vi "Teleop.vi"(10 "Match Info":T3={"Autonomous Elapsed Seconds"=0.0, "TeleOp Elapsed Seconds"=0.0, "Disabled Elapsed Seconds"=0.0, "Visited Autonomous"=FALSE, "Visited TeleOp"=FALSE, "Visited Disabled"=FALSE, "Autonomous Settings"={"Autonomous Style"=enum."Independent", "VI Refnum"=refnum}}, 11 "Call Context":T4) -> ()   [LabVIEW 2018]
doc: "This VI is called for each TeleOp packet received from the DS where the robot is not disabled. It is often used to read from the joysticks and update I/O or to update setpoints for timed control loops. It should complete and return within 20 milliseconds or it may miss DS packets."
uses:
  <vilib>/Rock Robotics/WPI/DriverStation/WPI_DriverStationDerivedRobotMode.ctl
  <vilib>/Rock Robotics/WPI/DriverStation/WPI_DriverStationMatch Info.ctl
  <vilib>/Rock Robotics/WPI/Utilities/WPI_GetSetVariantRefNum.vi
  <vilib>/Rock Robotics/Network Tables/NT Write Numeric Array.vi
  <vilib>/Rock Robotics/Network Tables/NT Read Boolean.vi
  <vilib>/Rock Robotics/Network Tables/NT Read Number.vi
  Robot Global Data.vi
  <vilib>/Rock Robotics/Network Tables/NT Write Boolean Array.vi
  <vilib>/addons/control/pid/pid.llb/PID (DBL).vi
  <vilib>/addons/control/pid/pid.llb/PID (DBL Array).vi
  <vilib>/Rock Robotics/WPI/Solenoid/Deprecated/WPI_SolenoidSetBool.vi
  <vilib>/addons/control/pid/NI_PID_pid.lvlib
panel:
  out "Distance 2":dbl
  in  "PID gains 4":T1={"proportional gain (Kc)"=1.0, "integral time (Ti, min)"=0.01, "derivative time (Td, min)"=0.0} {"derivative time (Td, min)" format="%.3f"; "integral time (Ti, min)" format="%.3f"; "proportional gain (Kc)" format="%.3f"}
  out "Direction 4":bool
  in  "Boolean":bool
  in  "PID gains 8":T1={"proportional gain (Kc)"=0.25, "integral time (Ti, min)"=0.001, "derivative time (Td, min)"=0.0}
  in  "PID gains":T2(array[cluster])=[{"proportional gain (Kc)"=1.0, "integral time (Ti, min)"=0.01, "derivative time (Td, min)"=0.0}] {"derivative time (Td, min)" format="%.3f"; "integral time (Ti, min)" format="%.3f"; "proportional gain (Kc)" format="%.3f"}
  in  "PID gains 2":T1={"proportional gain (Kc)"=1.0, "integral time (Ti, min)"=0.01, "derivative time (Td, min)"=0.0} {"derivative time (Td, min)" format="%.3f"; "integral time (Ti, min)" format="%.3f"; "proportional gain (Kc)" format="%.3f"}
  out "Compressor Running":bool
  out "Enable":bool
  out "Sample Slider 0":dbl(slide) scale=0.0..5.0
  out "Sample Boolean 1":bool
  out "Sample Boolean 0":bool
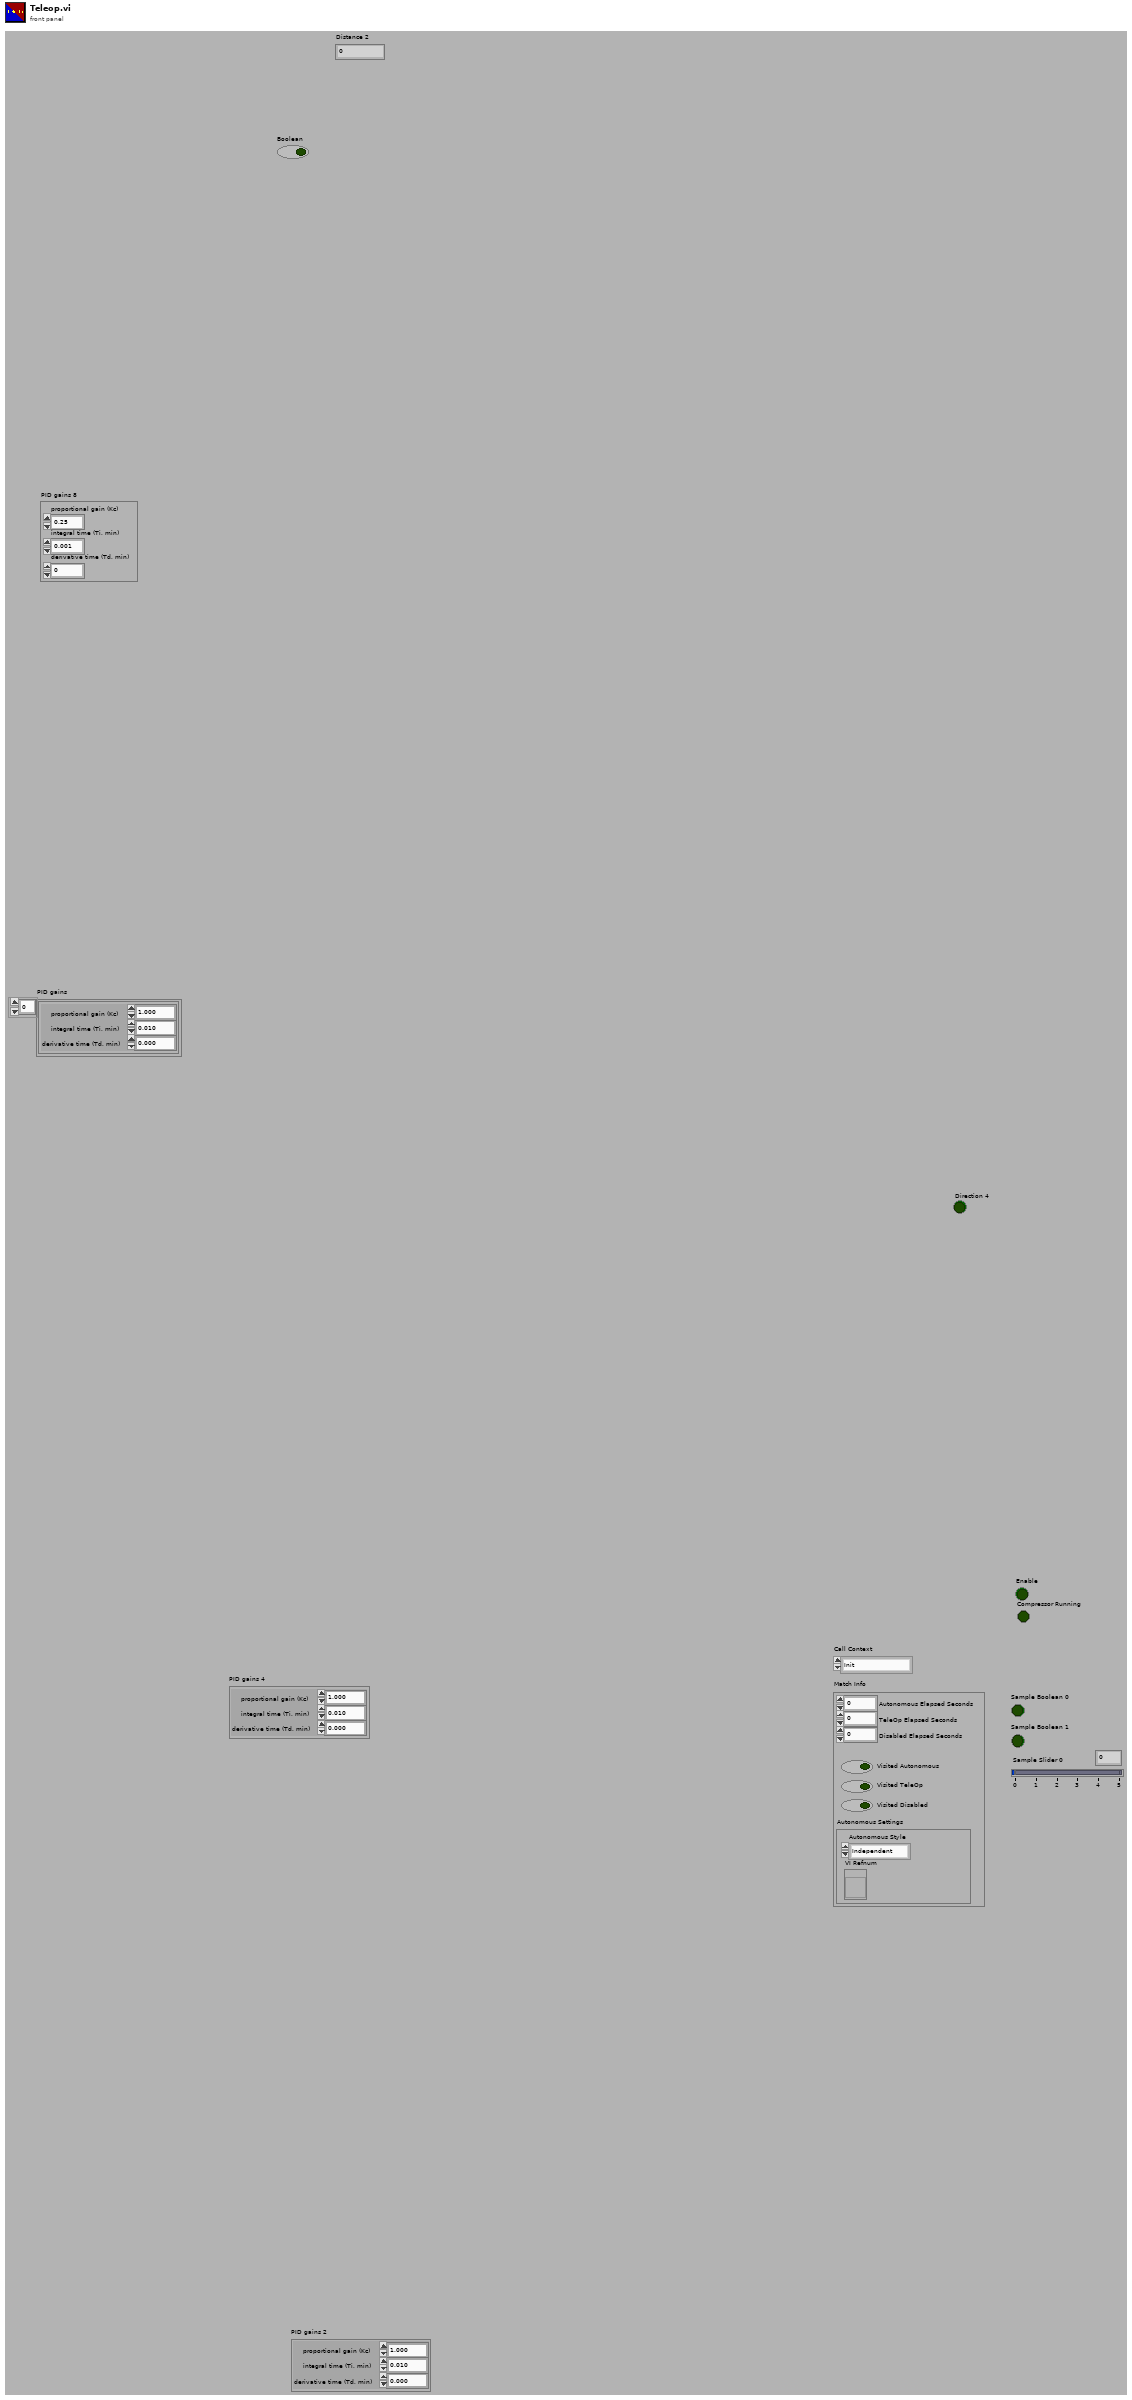
[diagram p1: front panel]
types:
  T1 = cluster{"proportional gain (Kc)":dbl, "integral time (Ti, min)":dbl, "derivative time (Td, min)":dbl}
  T2 = cluster{"proportional gain (Kc)":dbl, "integral time (Ti, min)":dbl, "derivative time (Td, min)":dbl}[]
  T3 = typedef "WPI_DriverStationMatch Info.ctl" = cluster{"Autonomous Elapsed Seconds":dbl, "TeleOp Elapsed Seconds":dbl, "Disabled Elapsed Seconds":dbl, "Visited Autonomous":bool, "Visited TeleOp":bool, "Visited Disabled":bool, "Autonomous Settings":cluster{"Autonomous Style":enum16{"Iterative", "Independent"}, "VI Refnum":refnum<vi>}}
  T4 = typedef "WPI_DriverStationDerivedRobotMode.ctl" = enum16{"Init", "Execute", "Stop"}
  T5 = enum16{"EXPULSA DISCO", "EXPULSA BOLA", "POSI敲O ENTREGA", "PEGAR BOLA", "POSI敲O NEUTRA", "DESCE ELEVADOR", "TERMINA SEQUENCIA"}[][]
  T6 = enum16{"EXPULSA DISCO", "EXPULSA BOLA", "POSI敲O ENTREGA", "PEGAR BOLA", "POSI敲O NEUTRA", "DESCE ELEVADOR", "TERMINA SEQUENCIA"}
  T7 = typedef "WPI_JoystickDevRef.ctl" = cluster{"Device":T8}
  T8 = typedef "WPI_JoystickDeviceEnum.ctl" = enum16{"USB 0", "USB 1", "USB 2", "USB 3", "USB 4", "USB 5"}
  T9 = typedef "WPI_EncoderDevRef.ctl" = cluster{"DevStatus":errorcluster, "EncoderIndex":T10, "CounterIndex":T11, "DistancePerCount":dbl, "Decoding Type":T12}
  T10 = typedef "FPGA_EncoderIdx.ctl" = enum8{"Enc 0", "Enc 1", "Enc 2", "Enc 3", "Enc 4", "Enc 5", "Enc 6", "Enc 7", "Invalid"}
  T11 = typedef "FPGA_CounterCtrSystemIndex.ctl" = enum8{"Ctr 0", "Ctr 1", "Ctr 2", "Ctr 3", "Ctr 4", "Ctr 5", "Ctr 6", "Ctr 7", "Invalid"}
  T12 = typedef "WPI_EncoderType.ctl" = enum16{"1x", "2x", "4x"}
  T13 = typedef "WPI_SolenoidDevRef.ctl" = cluster{"DevStatus":errorcluster, "Pneumatics Control Module":u8, "Forward Solenoid Channel":T14, "Reverse Solenoid Channel":T14}
  T14 = typedef "WPI_SolenoidChannel.ctl" = enum8{"Solenoid 0", "Solenoid 1", "Solenoid 2", "Solenoid 3", "Solenoid 4", "Solenoid 5", "Solenoid 6", "Solenoid 7", "Invalid"}
  T15 = typedef "WPI_DigitalInputDevRef.ctl" = cluster{"DevStatus":errorcluster, "DIO Channel":T16}
  T16 = typedef "FPGA_DIOChannel.ctl" = enum8{"DIO 0", "DIO 1", "DIO 2", "DIO 3", "DIO 4", "DIO 5", "DIO 6", "DIO 7", "DIO 8", "DIO 9", "DIO MXP 0", "DIO MXP 1", "DIO MXP 2", "DIO MXP 3", "DIO MXP 4", "DIO MXP 5", "DIO MXP 6", "DIO MXP 7", "DIO MXP 8", "DIO MXP 9", "DIO MXP 10", "DIO MXP 11", "DIO MXP 12", "DIO MXP 13", "DIO MXP 14", "DIO MXP 15", "SPI Port CS1", "SPI Port CS2", "SPI Port CS3", "SPI Port MISO", "SPI Port MOSI", "Invalid"}
  T17 = typedef "WPI_RobotDriveDevRef.ctl" = cluster{"DevStatus":errorcluster, "Motors[]":T18[], "Square Inputs":bool, "Max Output":dbl}
  T18 = typedef "WPI_MotorControlDeviceRef.ctl" = cluster{"DeviceStatus":errorcluster, "Type":T19, "PWM":cluster{"PWM Channel":T20, "DeadBand":T21}, "CAN":cluster{"Device Number":u8, "SetOutput VI Ref":variant, "GetOutput VI Ref":variant, "Enable VI Ref":variant, "Disable VI Ref":variant, "Data":variant}, "Invert":bool, "DIO PWM":cluster{"PWM \"Enable\" Channel":T20, "DIOChannel":T16, "PWM Rate":dbl}}
  T19 = typedef "WPI_MotorControlType.ctl" = enum16{"PWM", "CAN", "DIO PWM"}
  T20 = typedef "FPGA_DIOPWMChannel.ctl" = enum8{"PWM 0", "PWM 1", "PWM 2", "PWM 3", "PWM 4", "PWM 5", "PWM 6", "PWM 7", "PWM 8", "PWM 9", "PWM MXP 0", "PWM MXP 1", "PWM MXP 2", "PWM MXP 3", "PWM MXP 4", "PWM MXP 5", "PWM MXP 6", "PWM MXP 7", "PWM MXP 8", "PWM MXP 9", "Invalid"}
  T21 = typedef "WPI_PWMDeadband.ctl" = cluster{"Name":string, "maxPositivePwm":i32, "minPositivePwm":i32, "centerPwm":i32, "maxNegativePwm":i32, "minNegativePwm":i32, "angularRange":u16}
  T22 = typedef "WPI_CompressorDevRef.ctl" = cluster{"DevStatus":errorcluster, "Pneumatics Control Module":u8}
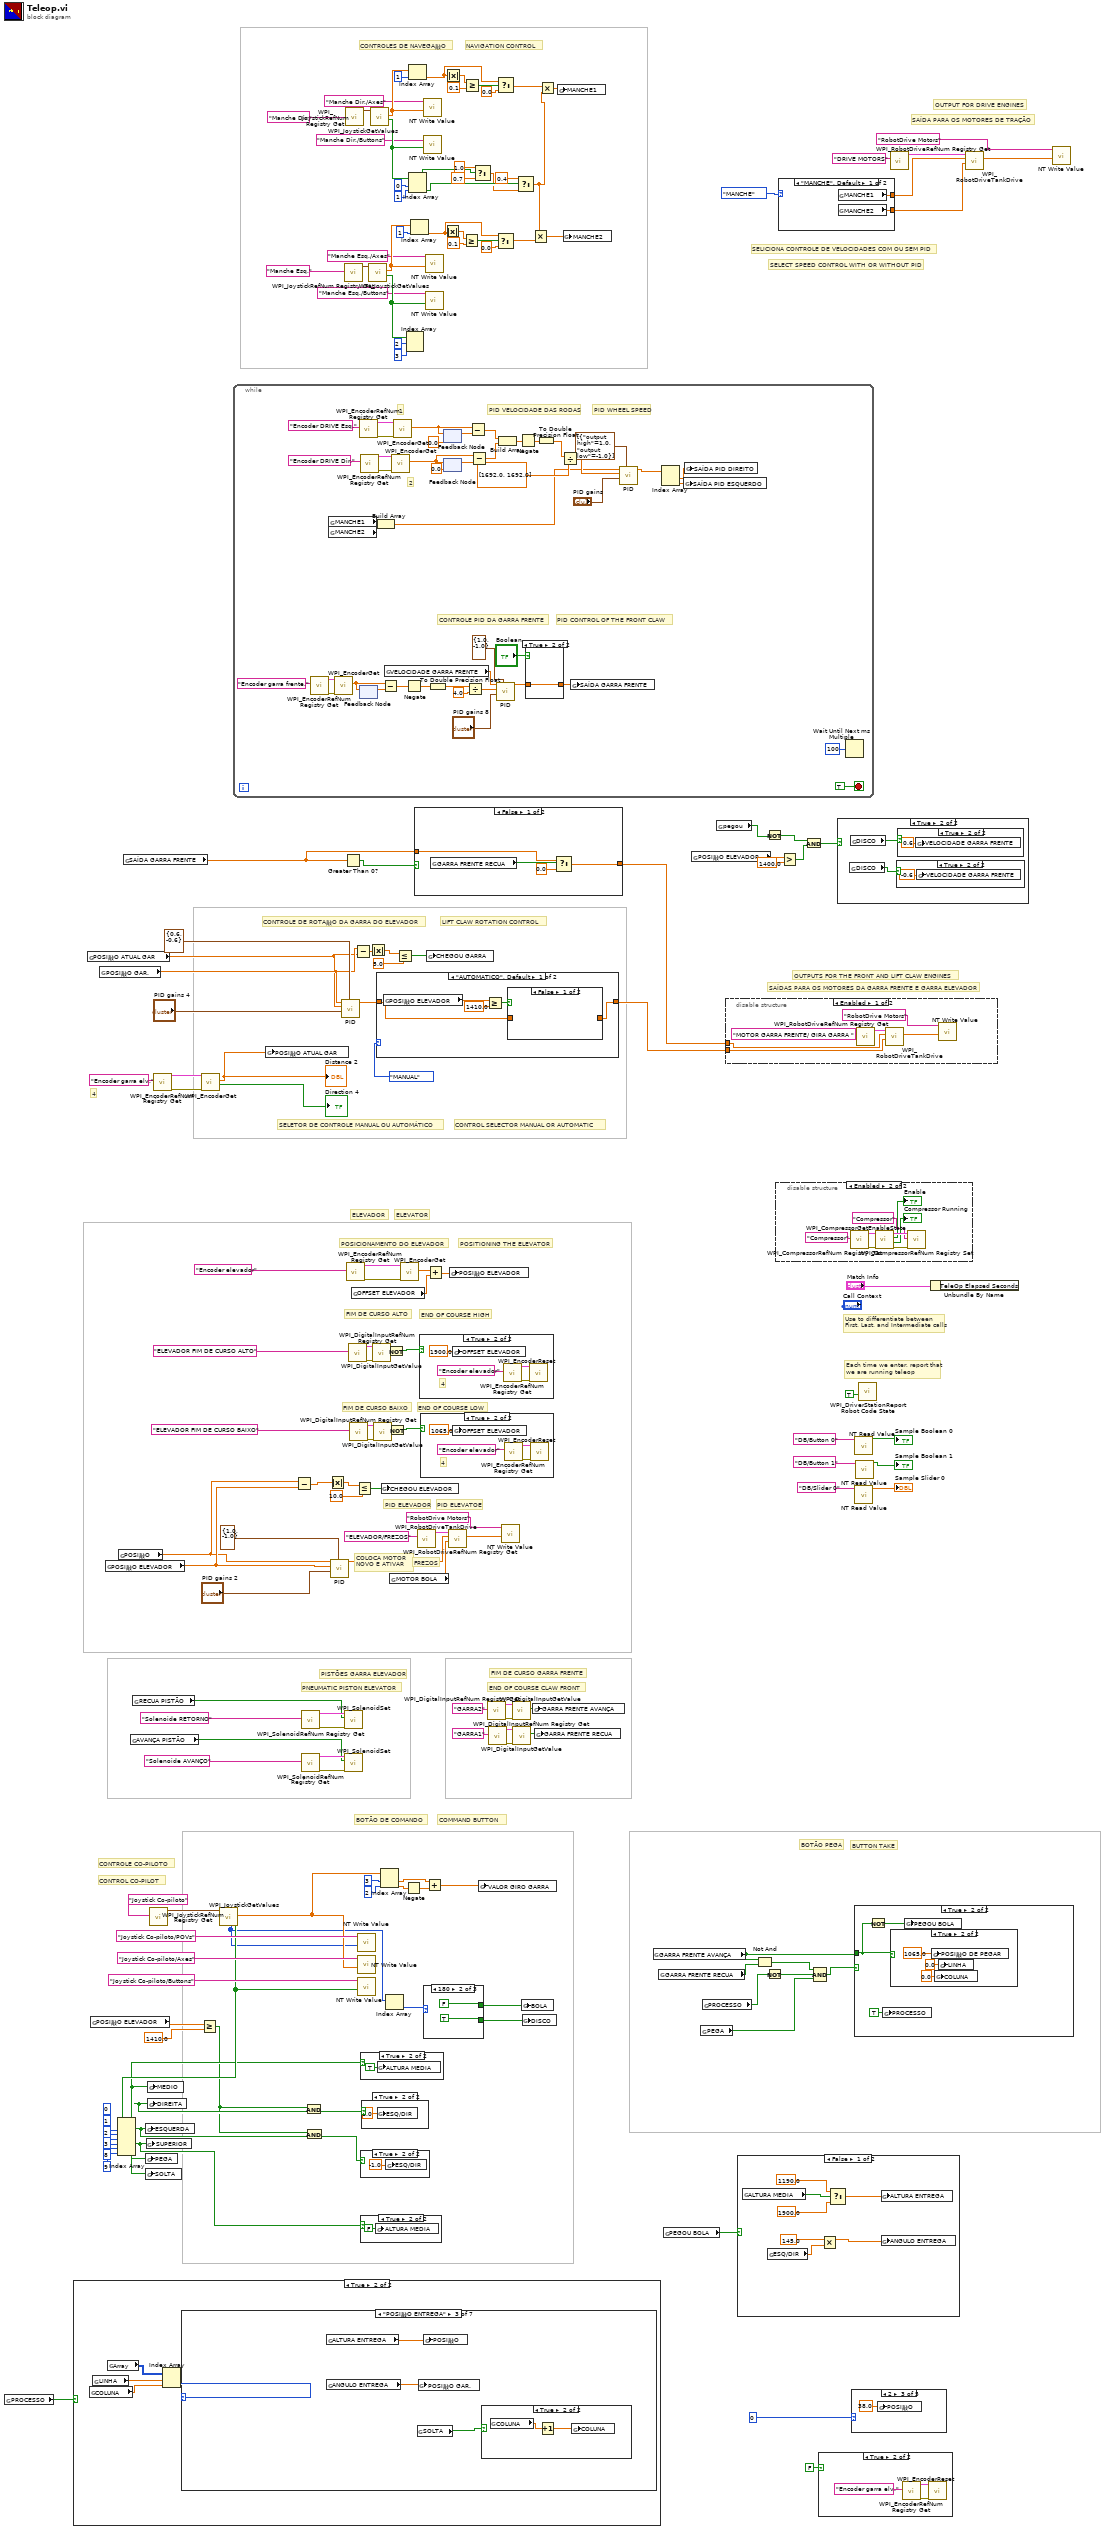
[diagram p0: block diagram]
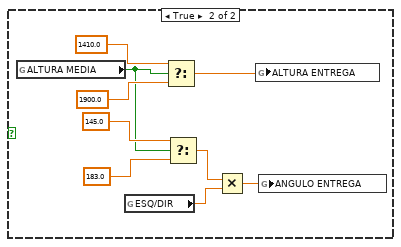
[diagram p6: hidden frame]
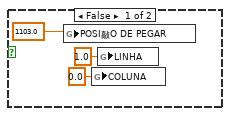
[diagram p8: hidden frame]
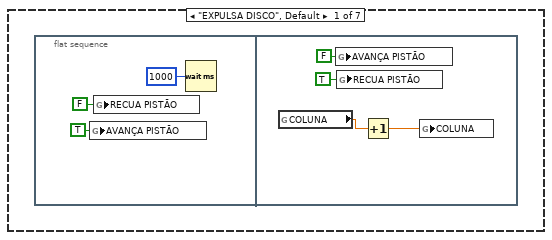
[diagram p10: hidden frame]
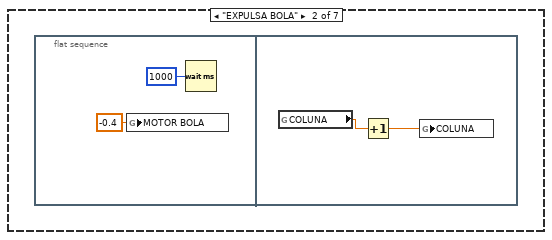
[diagram p11: hidden frame]
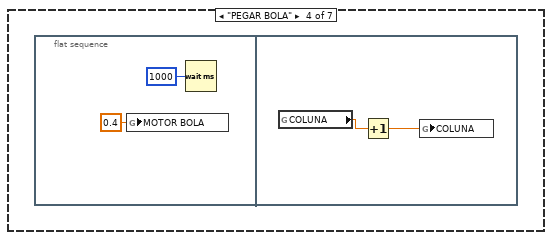
[diagram p13: hidden frame]
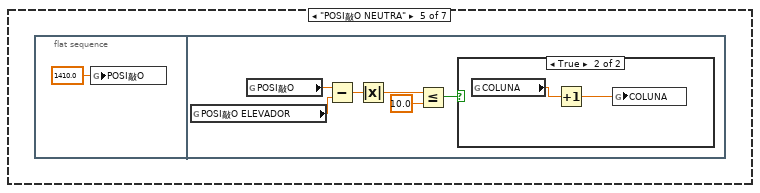
[diagram p14: hidden frame]
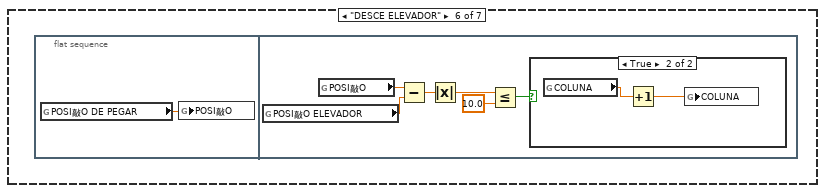
[diagram p16: hidden frame]
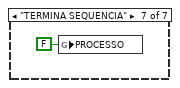
[diagram p18: hidden frame]
diagram:
  # "CONTROL CO-PILOT"
  # "BUTTON TAKE"
  # "COMMAND BUTTON"
  # "END OF COURSE CLAW FRONT"
  # "PNEUMATIC PISTON ELEVATOR"
  # "PID ELEVATOE"
  # "END OF COURSE LOW"
  # "END OF COURSE HIGH"
  # "ELEVATOR"
  # "POSITIONING THE ELEVATOR"
  # "CONTROL SELECTOR MANUAL OR AUTOMATIC"
  # "LIFT CLAW ROTATION CONTROL"
  # "OUTPUTS FOR THE FRONT AND LIFT CLAW ENGINES"
  # "SELECT SPEED CONTROL WITH OR WITHOUT PID"
  # "OUTPUT FOR DRIVE ENGINES"
  # "NAVIGATION CONTROL"
  # "FIM DE CURSO GARRA FRENTE"
  # "BOTÃO PEGA"
  # "BOTÃO DE COMANDO"
  # "FREZOS"
  # "FIM DE CURSO BAIXO"
  # "FIM DE CURSO ALTO"
  # "ELEVADOR"
  # "SAÍDAS PARA OS MOTORES DA GARRA FRENTE E GARRA ELEVADOR"
  # "SELETOR DE CONTROLE MANUAL OU AUTOMÁTICO"
  # "CONTROLE DE ROTA敲O DA GARRA DO ELEVADOR"
  # "SAÍDA PARA OS MOTORES DE TRAÇÃO"
  # "SELICIONA CONTROLE DE VELOCIDADES COM OU SEM PID"
  # "POSICIONAMENTO DO ELEVADOR"
  # "COLOCA MOTOR \nNOVO E ATIVAR"
  # "CONTROLE CO-PILOTO"
  # "PID ELEVADOR"
  # "4"
  # "CONTROLES DE NAVEGA敲O"
  # "PISTÕES GARRA ELEVADOR"
  # "Each time we enter, report that\nwe are running teleop"
  # "Use to differentiate between\nFirst, Last, and Intermediate calls"
  n1 = global read "Robot Global Data.vi" "PROCESSO"() -> (w27:bool)
  n2 = case shown="True" w27 {
    frame False {
    }
    frame True {
      n3 = global read "Robot Global Data.vi" "COLUNA"() -> (w172:dbl)
      n4 = global read "Robot Global Data.vi" "LINHA"() -> (w173:dbl)
      n5 = global read "Robot Global Data.vi" "Array"() -> (w174:T5)
      n6 = Index Array(array=w174, index (row)=w173, index (col)=w172) -> (element=w171:T6)
      n7 = case shown="\"POSI敲O ENTREGA\"" w171 {
        frame "EXPULSA DISCO", Default {
          n8 = flat-sequence {
            frame #0 {
              n9 = global write "Robot Global Data.vi" "AVANÇA PISTÃO"(TRUE ("AVANÇA PISTÃO")) -> ()
              n10 = global write "Robot Global Data.vi" "RECUA PISTÃO"(FALSE ("RECUA PISTÃO")) -> ()
              n11 = Wait (ms)(milliseconds to wait=u32 1000) -> ()  [unwired: 1 out]
            }
            frame #1 {
              n12 = global read "Robot Global Data.vi" "COLUNA"() -> (w181:dbl)
              n13 = global write "Robot Global Data.vi" "AVANÇA PISTÃO"(FALSE ("AVANÇA PISTÃO")) -> ()
              n14 = global write "Robot Global Data.vi" "RECUA PISTÃO"(TRUE ("RECUA PISTÃO")) -> ()
              n15 = Increment(x=w181) -> (x+1=w180:dbl)
              n16 = global write "Robot Global Data.vi" "COLUNA"(w180) -> ()
            }
          }
        }
        frame "EXPULSA BOLA" {
          n17 = flat-sequence {
            frame #0 {
              n18 = global write "Robot Global Data.vi" "MOTOR BOLA"(-0.4 ("MOTOR BOLA")) -> ()
              n19 = Wait (ms)(milliseconds to wait=u32 1000) -> ()  [unwired: 1 out]
            }
            frame #1 {
              n20 = global read "Robot Global Data.vi" "COLUNA"() -> (w185:dbl)
              n21 = Increment(x=w185) -> (x+1=w184:dbl)
              n22 = global write "Robot Global Data.vi" "COLUNA"(w184) -> ()
            }
          }
        }
        frame "POSI敲O ENTREGA" {
          n23 = global read "Robot Global Data.vi" "ALTURA ENTREGA"() -> (w188:dbl)
          n24 = global read "Robot Global Data.vi" "ANGULO ENTREGA"() -> (w187:dbl)
          n25 = global read "Robot Global Data.vi" "SOLTA"() -> (w186:bool)
          n26 = global write "Robot Global Data.vi" "POSI敲O GAR."(w187) -> ()
          n27 = global write "Robot Global Data.vi" "POSI敲O"(w188) -> ()
          n28 = case shown="True" w186 {
            frame False {
            }
            frame True {
              n29 = global read "Robot Global Data.vi" "COLUNA"() -> (w190:dbl)
              n30 = Increment(x=w190) -> (x+1=w189:dbl)
              n31 = global write "Robot Global Data.vi" "COLUNA"(w189) -> ()
            }
          }
        }
        frame "PEGAR BOLA" {
          n32 = flat-sequence {
            frame #0 {
              n33 = global write "Robot Global Data.vi" "MOTOR BOLA"(0.4 ("MOTOR BOLA")) -> ()
              n34 = Wait (ms)(milliseconds to wait=u32 1000) -> ()  [unwired: 1 out]
            }
            frame #1 {
              n35 = global read "Robot Global Data.vi" "COLUNA"() -> (w194:dbl)
              n36 = Increment(x=w194) -> (x+1=w193:dbl)
              n37 = global write "Robot Global Data.vi" "COLUNA"(w193) -> ()
            }
          }
        }
        frame "POSI敲O NEUTRA" {
          n38 = flat-sequence {
            frame #0 {
              n39 = global write "Robot Global Data.vi" "POSI敲O"(1410.0 ("POSI敲O")) -> ()
            }
            frame #1 {
              n40 = global read "Robot Global Data.vi" "POSI敲O ELEVADOR"() -> (w197:dbl)
              n41 = global read "Robot Global Data.vi" "POSI敲O"() -> (w199:dbl)
              n42 = Subtract(x=w199, y=w197) -> (x-y=w198:dbl)
              n43 = Absolute Value(x=w198) -> (abs(x)=w200:dbl)
              n44 = Less Or Equal?(x=w200, y=10.0) -> (x <= y?=w201:bool)
              n45 = case shown="True" w201 {
                frame False {
                }
                frame True {
                  n46 = global read "Robot Global Data.vi" "COLUNA"() -> (w203:dbl)
                  n47 = Increment(x=w203) -> (x+1=w202:dbl)
                  n48 = global write "Robot Global Data.vi" "COLUNA"(w202) -> ()
                }
              }
            }
          }
        }
        frame "DESCE ELEVADOR" {
          n49 = flat-sequence {
            frame #0 {
              n50 = global read "Robot Global Data.vi" "POSI敲O DE PEGAR"() -> (w204:dbl)
              n51 = global write "Robot Global Data.vi" "POSI敲O"(w204) -> ()
            }
            frame #1 {
              n52 = global read "Robot Global Data.vi" "POSI敲O ELEVADOR"() -> (w206:dbl)
              n53 = global read "Robot Global Data.vi" "POSI敲O"() -> (w208:dbl)
              n54 = Subtract(x=w208, y=w206) -> (x-y=w207:dbl)
              n55 = Absolute Value(x=w207) -> (abs(x)=w209:dbl)
              n56 = Less Or Equal?(x=w209, y=10.0) -> (x <= y?=w210:bool)
              n57 = case shown="True" w210 {
                frame False {
                }
                frame True {
                  n58 = global read "Robot Global Data.vi" "COLUNA"() -> (w212:dbl)
                  n59 = Increment(x=w212) -> (x+1=w211:dbl)
                  n60 = global write "Robot Global Data.vi" "COLUNA"(w211) -> ()
                }
              }
            }
          }
        }
        frame "TERMINA SEQUENCIA" {
          n61 = global write "Robot Global Data.vi" "PROCESSO"(FALSE ("PROCESSO")) -> ()
        }
      }
    }
  }
  n62 = global read "Robot Global Data.vi" "POSI敲O ATUAL GAR"() -> (w28:dbl)
  n63 = global read "Robot Global Data.vi" "POSI敲O ELEVADOR"() -> (w6:dbl)
  n64 = global read "Robot Global Data.vi" "POSI敲O GAR."() -> (w39:dbl)
  n65 = global read "Robot Global Data.vi" "POSI敲O ELEVADOR"() -> (w31:dbl)
  n66 = global read "Robot Global Data.vi" "POSI敲O"() -> (w30:dbl)
  n67 = global read "Robot Global Data.vi" "SAÍDA GARRA FRENTE"() -> (w137:dbl)
  n68 = global read "Robot Global Data.vi" "AVANÇA PISTÃO"() -> (w55:bool)
  n69 = global read "Robot Global Data.vi" "RECUA PISTÃO"() -> (w56:bool)
  n70 = call <vilib>:"WPI_JoystickRefNum Registry Get.vi"("refnum name"="Joystick Co-piloto") -> ("JoystickDevRef"=w155:T7)  [unwired: 1 in, 9 out]
  n71 = call <vilib>:"WPI_EncoderRefNum Registry Get.vi"("refnum name"="Encoder garra elv.") -> ("error out"=w131:errorcluster, "EncoderDevRef"=w132:T9)  [unwired: 9 in]
  n72 = Greater Or Equal?(x=w6, y=1410.0) -> (x >= y?=w2:bool)
  n73 = call <vilib>:"WPI_EncoderGet.vi"("error in (no error)"=w131, "EncoderDevRef"=w132) -> ("Direction"=→"Direction 4":bool, "Distance"=w29:dbl)  [unwired: 4 in, 4 out]
  "Distance 2" <- w29
  n74 = call <vilib>:"WPI_JoystickGetValues.vi"("JoystickDevRef"=w155) -> ("Buttons"=w129:bool[], "Axes"=w139:dbl[], "POVs"=w50:i16[])  [unwired: 6 in, 2 out]
  n75 = Index Array(array=w129, index #1=0 ("index"), index #2=1 ("index"), index #3=2 ("index"), index #4=3 ("index"), index #5=8 ("index"), index #6=9 ("index")) -> (element #1=w10:bool, element #2=w9:bool, element #3=w8:bool, element #4=w7:bool, element #5=w54:bool, element #6=w53:bool)
  n76 = global write "Robot Global Data.vi" "ESQUERDA"(w8) -> ()
  n77 = global write "Robot Global Data.vi" "PEGA"(w54) -> ()
  n78 = global write "Robot Global Data.vi" "SOLTA"(w53) -> ()
  n79 = global write "Robot Global Data.vi" "SUPERIOR"(w7) -> ()
  n80 = global write "Robot Global Data.vi" "MEDIO"(w10) -> ()
  n81 = global write "Robot Global Data.vi" "DIREITA"(w9) -> ()
  n82 = while {
    stop <- TRUE stop-if-true
    # "PID CONTROL OF THE FRONT CLAW"
    # "PID WHEEL SPEED"
    # "PID VELOCIDADE DAS RODAS"
    # "2"
    # "1"
    # "CONTROLE PID DA GARRA FRENTE"
    n83 = call <vilib>:"WPI_EncoderRefNum Registry Get.vi"("refnum name"="Encoder garra frente.") -> ("error out"=w255:errorcluster, "EncoderDevRef"=w254:T9)  [unwired: 9 in]
    n84 = global read "Robot Global Data.vi" "MANCHE1"() -> (w225:dbl)
    n85 = global read "Robot Global Data.vi" "MANCHE2"() -> (w226:dbl)
    n86 = call <vilib>:"WPI_EncoderGet.vi"("error in (no error)"=w255, "EncoderDevRef"=w254) -> ("Distance"=w253:dbl)  [unwired: 4 in, 5 out]
    n87 = call <vilib>:"WPI_EncoderRefNum Registry Get.vi"("refnum name"="Encoder DRIVE Esq.") -> ("error out"=w230:errorcluster, "EncoderDevRef"=w231:T9)  [unwired: 9 in]
    n88 = feedback #1() -> (w256:dbl)  [unwired: 1 in]
    n89 = feedback-in #1(w253) -> ()
    n90 = call <vilib>:"WPI_EncoderRefNum Registry Get.vi"("refnum name"="Encoder DRIVE Dir.") -> ("error out"=w233:errorcluster, "EncoderDevRef"=w234:T9)  [unwired: 9 in]
    n91 = Build Array(w225, w226) -> (w227:dbl[])
    n92 = Subtract(x=w253, y=w256) -> (x-y=w250:dbl)
    n93 = global read "Robot Global Data.vi" "VELOCIDADE GARRA FRENTE"() -> (w245:dbl)
    n94 = call <vilib>:"WPI_EncoderGet.vi"("error in (no error)"=w233, "EncoderDevRef"=w234) -> ("Distance"=w235:dbl)  [unwired: 4 in, 5 out]
    n95 = call <vilib>:"WPI_EncoderGet.vi"("error in (no error)"=w230, "EncoderDevRef"=w231) -> ("Distance"=w232:dbl)  [unwired: 4 in, 5 out]
    n96 = Negate(x=w250) -> (-x=w251:dbl)
    n97 = To Double Precision Float(number=w251) -> (double precision float=w249:dbl)
    n98 = feedback #2(0.0 ("Distance")) -> (w219:dbl)
    n99 = feedback-in #2(w232) -> ()
    n100 = feedback #3(0.0 ("Distance")) -> (w222:dbl)
    n101 = feedback-in #3(w235) -> ()
    n102 = Divide(x=w249, y=4.0) -> (x/y=w247:dbl)
    n103 = Subtract(x=w232, y=w219) -> (x-y=w223:dbl)
    n104 = Subtract(x=w235, y=w222) -> (x-y=w224:dbl)
    n105 = call-poly <vilib>:"PID.vi"("output range"=cluster{"output high":dbl, "output low":dbl} {"output high"=1.0, "output low"=-1.0}, "PID gains"="PID gains 8", "process variable"=w247, "setpoint"=w245) -> ("output"=w243:dbl)  [unwired: 6 in, 1 out]
    n106 = Build Array(w223, w224) -> (w217:dbl[])
    n107 = Negate(x=w217) -> (-x=w218:dbl[])
    n108 = case shown="True" "Boolean" {
      tunnel: w243 -> [_ w259]
      tunnel: [_ w259] -> w242
      frame False {
      }
      frame True {
      }
    }
    n109 = To Double Precision Float(number=w218) -> (double precision float=w239:dbl[])
    n110 = Divide(x=w239, y=dbl[] [1692.0, 1692.0]) -> (x/y=w240:dbl[])
    n111 = global write "Robot Global Data.vi" "SAÍDA GARRA FRENTE"(w242) -> ()
    n112 = call-poly <vilib>:"PID.vi"("output range"=cluster{"output high":dbl, "output low":dbl}[] [{"output high"=1.0, "output low"=-1.0}], "PID gains"="PID gains", "process variable"=w240, "setpoint"=w227) -> ("output"=w216:dbl[])  [unwired: 6 in, 1 out]
    n113 = Index Array(array=w216) -> (element #1=w215:dbl, element #2=w214:dbl)  [unwired: 2 in]
    n114 = global write "Robot Global Data.vi" "SAÍDA PID ESQUERDO"(w214) -> ()
    n115 = global write "Robot Global Data.vi" "SAÍDA PID DIREITO"(w215) -> ()
    n116 = Wait Until Next ms Multiple(millisecond multiple=u32 100) -> ()  [unwired: 1 out]
  }
  n117 = global write "Robot Global Data.vi" "POSI敲O ATUAL GAR"(w29) -> ()
  n118 = Subtract(x=w30, y=w31) -> (x-y=w35:dbl)
  n119 = call <vilib>:"WPI_SolenoidRefNum Registry Get.vi"("refnum name"="Solenoide RETORNO") -> ("error out"=w114:errorcluster, "SolenoidDevRef"=w119:T13)  [unwired: 9 in]
  n120 = call <vilib>:"WPI_SolenoidRefNum Registry Get.vi"("refnum name"="Solenoide AVANÇO") -> ("error out"=w117:errorcluster, "SolenoidDevRef"=w116:T13)  [unwired: 9 in]
  n121 = And(x=w2, y=w9) -> (x .and. y?=w4:bool)
  n122 = And(x=w2, y=w8) -> (x .and. y?=w3:bool)
  n123 = Absolute Value(x=w35) -> (abs(x)=w34:dbl)
  n124 = call-poly <vilib>:"PID.vi"("output range"=cluster{"output high":dbl, "output low":dbl} {"output high"=1.0, "output low"=-1.0}, "PID gains"="PID gains 2", "process variable"=w31, "setpoint"=w30) -> ("output"=w57:dbl)  [unwired: 6 in, 1 out]
  n125 = call-poly <vilib>:"PID.vi"("output range"=cluster{"output high":dbl, "output low":dbl} {"output high"=0.6, "output low"=-0.6}, "PID gains"="PID gains 4", "process variable"=w28, "setpoint"=w39) -> ("output"=w97:dbl)  [unwired: 6 in, 1 out]
  n126 = Greater Than 0?(x=w137) -> (x > 0?=w138:bool)
  n127 = call <vilib>:"WPI_JoystickRefNum Registry Get.vi"("refnum name"="Manche Esq.") -> ("JoystickDevRef"=w160:T7)  [unwired: 1 in, 9 out]
  n128 = call-poly <vilib>:"WPI_SolenoidSet.vi"("error in (no error)"=w114, "Value"=w56, "SolenoidDevRef"=w119) -> ()  [unwired: 7 in, 2 out]
  n129 = call-poly <vilib>:"WPI_SolenoidSet.vi"("error in (no error)"=w117, "Value"=w55, "SolenoidDevRef"=w116) -> ()  [unwired: 7 in, 2 out]
  n130 = call <vilib>:"WPI_JoystickRefNum Registry Get.vi"("refnum name"="Manche Dir.") -> ("JoystickDevRef"=w149:T7)  [unwired: 1 in, 9 out]
  n131 = call <vilib>:"WPI_EncoderRefNum Registry Get.vi"("refnum name"="Encoder elevador") -> ("error out"=w144:errorcluster, "EncoderDevRef"=w143:T9)  [unwired: 9 in]
  n132 = call <vilib>:"WPI_DigitalInputRefNum Registry Get.vi"("refnum name"="ELEVADOR FIM DE CURSO ALTO") -> ("error out"=w108:errorcluster, "DigitalInputDevRef"=w106:T15)  [unwired: 9 in]
  n133 = call <vilib>:"WPI_DigitalInputRefNum Registry Get.vi"("refnum name"="ELEVADOR FIM DE CURSO BAIXO") -> ("error out"=w103:errorcluster, "DigitalInputDevRef"=w105:T15)  [unwired: 9 in]
  n134 = global read "Robot Global Data.vi" "OFFSET ELEVADOR"() -> (w111:dbl)
  n135 = Subtract(x=w39, y=w28) -> (x-y=w40:dbl)
  n136 = Less Or Equal?(x=w34, y=10.0) -> (x <= y?=w32:bool)
  n137 = call-poly <vilib>:"NT Write Value.vi"("Numeric Array"=w50, "Name"="Joystick Co-piloto/POVs") -> ()  [unwired: 9 in, 1 out]
  n138 = call-poly <vilib>:"NT Write Value.vi"("Numeric Array"=w139, "Name"="Joystick Co-piloto/Axes") -> ()  [unwired: 9 in, 1 out]
  n139 = call-poly <vilib>:"NT Write Value.vi"("Boolean Array"=w129, "Name"="Joystick Co-piloto/Buttons") -> ()  [unwired: 9 in, 1 out]
  n140 = case shown="True" w3 {
    frame False {
    }
    frame True {
      n141 = global write "Robot Global Data.vi" "ESQ/DIR"(-1.0 ("ESQ/DIR")) -> ()
    }
  }
  n142 = case shown="True" w10 {
    frame False {
    }
    frame True {
      n143 = global write "Robot Global Data.vi" "ALTURA MEDIA"(TRUE ("ALTURA MEDIA")) -> ()
    }
  }
  n144 = case shown="True" w7 {
    frame False {
    }
    frame True {
      n145 = global write "Robot Global Data.vi" "ALTURA MEDIA"(FALSE ("ALTURA MEDIA")) -> ()
    }
  }
  n146 = case shown="True" w4 {
    frame False {
    }
    frame True {
      n147 = global write "Robot Global Data.vi" "ESQ/DIR"(1.0 ("ESQ/DIR")) -> ()
    }
  }
  n148 = call <vilib>:"WPI_JoystickGetValues.vi"("JoystickDevRef"=w160) -> ("Buttons"=w123:bool[], "Axes"=w168:dbl[])  [unwired: 6 in, 3 out]
  n149 = Absolute Value(x=w40) -> (abs(x)=w38:dbl)
  n150 = call <vilib>:"WPI_JoystickGetValues.vi"("JoystickDevRef"=w149) -> ("Buttons"=w120:bool[], "Axes"=w140:dbl[])  [unwired: 6 in, 3 out]
  n151 = call <vilib>:"WPI_DigitalInputGetValue.vi"("error in (no error)"=w108, "DigitalInputDevRef"=w106) -> ("Value"=w102:bool)  [unwired: 7 in, 2 out]
  n152 = call <vilib>:"WPI_DigitalInputGetValue.vi"("error in (no error)"=w103, "DigitalInputDevRef"=w105) -> ("Value"=w101:bool)  [unwired: 7 in, 2 out]
  n153 = case shown="\"AUTOMATICO\", Default" enum16{"AUTOMATICO", "MANUAL"}."MANUAL" {
    tunnel: w97 -> [w265 _]
    tunnel: [w264 w273] -> w1
    frame "AUTOMATICO", Default {
      n154 = global read "Robot Global Data.vi" "POSI敲O ELEVADOR"() -> (w268:dbl)
      n155 = Greater Or Equal?(x=w268, y=1410.0) -> (x >= y?=w266:bool)
      n156 = case shown="False" w266 {
        tunnel: [_ w269] -> w264
        tunnel: w265 -> [_ w269]
        frame False {
        }
        frame True {
        }
      }
    }
    frame "MANUAL" {
      n157 = global read "Robot Global Data.vi" "POSI敲O ELEVADOR"() -> (w272:dbl)
      n158 = Greater Or Equal?(x=w272, y=1410.0) -> (x >= y?=w270:bool)
      n159 = case shown="True" w270 {
        tunnel: [_ w274] -> w273
        frame False {
        }
        frame True {
          n160 = global read "Robot Global Data.vi" "VALOR GIRO GARRA"() -> (w274:dbl)
        }
      }
    }
  }
  n161 = Index Array(array=w139, index #1=3, index #2=2 ("index")) -> (element #1=w96:dbl, element #2=w95:dbl)
  n162 = global write "Robot Global Data.vi" "CHEGOU ELEVADOR"(w32) -> ()
  n163 = Index Array(array=w50) -> (element=w49:i16)  [unwired: 1 in]
  n164 = Not(x=w102) -> (.not. x?=w100:bool)
  n165 = Not(x=w101) -> (.not. x?=w99:bool)
  n166 = global read "Robot Global Data.vi" "MOTOR BOLA"() -> (w58:dbl)
  n167 = Less Or Equal?(x=w38, y=5.0) -> (x <= y?=w36:bool)
  n168 = call <vilib>:"WPI_EncoderGet.vi"("error in (no error)"=w144, "EncoderDevRef"=w143) -> ("Distance"=w112:dbl)  [unwired: 4 in, 5 out]
  n169 = Negate(x=w95) -> (-x=w94:dbl)
  n170 = Index Array(array=w123, index #1=2 ("index"), index #2=3 ("index")) -> ()  [unwired: 2 out]
  n171 = Index Array(array=w140, index=1) -> (element=w89:dbl)
  n172 = Index Array(array=w120, index #1=0 ("index"), index #2=1 ("index")) -> (element #1=w77:bool, element #2=w80:bool)
  n173 = Index Array(array=w168, index=1) -> (element=w81:dbl)
  n174 = case shown="False" w138 {
    tunnel: w137 -> [w278 w282]
    tunnel: [w276 w281] -> w136
    frame False {
      n175 = global read "Robot Global Data.vi" "GARRA FRENTE RECUA"() -> (w275:bool)
      n176 = Select(t=w278, s=w275, f=0.0) -> (s? t:f=w276:dbl)
    }
    frame True {
      n177 = global read "Robot Global Data.vi" "GARRA FRENTE AVANÇA"() -> (w279:bool)
      n178 = Not(x=w279) -> (.not. x?=w280:bool)
      n179 = global write "Robot Global Data.vi" "VELOCIDADE ZERO"(w280) -> ()
      n180 = Select(t=w282, s=w279, f=0.0) -> (s? t:f=w281:dbl)
    }
  }
  n181 = call <vilib>:"WPI_RobotDriveRefNum Registry Get.vi"("refnum name"="ELEVADOR/FREZOS") -> ("RobotDriveDevRef"=w61:T17)  [unwired: 1 in, 9 out]
  n182 = case shown="True" w100 {
    frame False {
    }
    frame True {
      # "4"
      n183 = global write "Robot Global Data.vi" "OFFSET ELEVADOR"(1900.0 ("OFFSET ELEVADOR")) -> ()
      n184 = call <vilib>:"WPI_EncoderRefNum Registry Get.vi"("refnum name"="Encoder elevador") -> ("error out"=w286:errorcluster, "EncoderDevRef"=w285:T9)  [unwired: 9 in]
      n185 = call <vilib>:"WPI_EncoderReset.vi"("error in (no error)"=w286, "EncoderDevRef"=w285) -> ()  [unwired: 8 in, 2 out]
    }
  }
  n186 = case shown="True" w99 {
    frame False {
    }
    frame True {
      # "4"
      n187 = global write "Robot Global Data.vi" "OFFSET ELEVADOR"(1065.0 ("OFFSET ELEVADOR")) -> ()
      n188 = call <vilib>:"WPI_EncoderRefNum Registry Get.vi"("refnum name"="Encoder elevador") -> ("error out"=w290:errorcluster, "EncoderDevRef"=w289:T9)  [unwired: 9 in]
      n189 = call <vilib>:"WPI_EncoderReset.vi"("error in (no error)"=w290, "EncoderDevRef"=w289) -> ()  [unwired: 8 in, 2 out]
    }
  }
  n190 = call-poly <vilib>:"NT Write Value.vi"("Numeric Array"=w140, "Name"="Manche Dir./Axes") -> ()  [unwired: 9 in, 1 out]
  n191 = call-poly <vilib>:"NT Write Value.vi"("Boolean Array"=w120, "Name"="Manche Dir./Buttons") -> ()  [unwired: 9 in, 1 out]
  n192 = case shown="180" w49 {
    tunnel: [TRUE ("BOLA") FALSE ("BOLA") _] -> w48
    tunnel: [FALSE ("BOLA") TRUE ("BOLA") _] -> w47
    frame 0 {
    }
    frame 180 {
    }
    frame -1, Default {
    }
  }
  n193 = call-poly <vilib>:"NT Write Value.vi"("Numeric Array"=w168, "Name"="Manche Esq./Axes") -> ()  [unwired: 9 in, 1 out]
  n194 = call-poly <vilib>:"NT Write Value.vi"("Boolean Array"=w123, "Name"="Manche Esq./Buttons") -> ()  [unwired: 9 in, 1 out]
  n195 = Add(x=w96, y=w94) -> (x+y=w93:dbl)
  n196 = global write "Robot Global Data.vi" "CHEGOU GARRA"(w36) -> ()
  n197 = Add(x=w112, y=w111) -> (x+y=w110:dbl)
  n198 = Absolute Value(x=w81) -> (abs(x)=w83:dbl)
  n199 = Absolute Value(x=w89) -> (abs(x)=w92:dbl)
  n200 = call <vilib>:"WPI_RobotDriveTankDrive.vi"("Right axis value"=w58, "Left axis value"=w57, "RobotDriveDevRef"=w61) -> ("Motor Values"=w59:dbl[])  [unwired: 6 in, 2 out]
  n201 = global write "Robot Global Data.vi" "POSI敲O ELEVADOR"(w110) -> ()
  n202 = Greater Or Equal?(x=w83, y=0.1) -> (x >= y?=w85:bool)
  n203 = Greater Or Equal?(x=w92, y=0.1) -> (x >= y?=w90:bool)
  n204 = Select(t=1.0, s=w77, f=0.7) -> (s? t:f=w78:dbl)
  n205 = global write "Robot Global Data.vi" "VALOR GIRO GARRA"(w93) -> ()
  n206 = call <vilib>:"WPI_DigitalInputRefNum Registry Get.vi"("refnum name"="GARRA2") -> ("error out"=w25:errorcluster, "DigitalInputDevRef"=w26:T15)  [unwired: 9 in]
  n207 = call <vilib>:"WPI_DigitalInputRefNum Registry Get.vi"("refnum name"="GARRA1") -> ("error out"=w22:errorcluster, "DigitalInputDevRef"=w19:T15)  [unwired: 9 in]
  n208 = Select(t=w81, s=w85, f=0.0) -> (s? t:f=w82:dbl)
  n209 = Select(t=w89, s=w90, f=0.0) -> (s? t:f=w87:dbl)
  n210 = call-poly <vilib>:"NT Write Value.vi"("Numeric Array"=w59, "Name"="RobotDrive Motors") -> ()  [unwired: 9 in, 1 out]
  n211 = call <vilib>:"WPI_DigitalInputGetValue.vi"("error in (no error)"=w25, "DigitalInputDevRef"=w26) -> ("Value"=w23:bool)  [unwired: 7 in, 2 out]
  n212 = call <vilib>:"WPI_DigitalInputGetValue.vi"("error in (no error)"=w22, "DigitalInputDevRef"=w19) -> ("Value"=w21:bool)  [unwired: 7 in, 2 out]
  n213 = Select(t=0.4, s=w80, f=w78) -> (s? t:f=w72:dbl)
  n214 = global write "Robot Global Data.vi" "BOLA"(w48) -> ()
  n215 = global write "Robot Global Data.vi" "DISCO"(w47) -> ()
  n216 = Multiply(x=w72, y=w82) -> (x*y=w73:dbl)
  n217 = global write "Robot Global Data.vi" "GARRA FRENTE AVANÇA"(w23) -> ()
  n218 = global write "Robot Global Data.vi" "GARRA FRENTE RECUA"(w21) -> ()
  n219 = Multiply(x=w87, y=w72) -> (x*y=w74:dbl)
  n220 = global write "Robot Global Data.vi" "MANCHE1"(w74) -> ()
  n221 = global write "Robot Global Data.vi" "MANCHE2"(w73) -> ()
  n222 = global read "Robot Global Data.vi" "GARRA FRENTE AVANÇA"() -> (w12:bool)
  n223 = global read "Robot Global Data.vi" "GARRA FRENTE RECUA"() -> (w18:bool)
  n224 = global read "Robot Global Data.vi" "PEGOU BOLA"() -> (w11:bool)
  n225 = global read "Robot Global Data.vi" "POSI敲O ELEVADOR"() -> (w46:dbl)
  n226 = global read "Robot Global Data.vi" "PEGA"() -> (w14:bool)
  n227 = global read "Robot Global Data.vi" "PROCESSO"() -> (w16:bool)
  n228 = global read "Robot Global Data.vi" "pegou"() -> (w43:bool)
  n229 = disable-structure shown="Enabled" {
    disable-tunnel: w136 -> [w297 _]
    disable-tunnel: w1 -> [w296 _]
    frame Enabled {
      n230 = call <vilib>:"WPI_RobotDriveRefNum Registry Get.vi"("refnum name"="MOTOR GARRA FRENTE/ GIRA GARRA ") -> ("RobotDriveDevRef"=w301:T17)  [unwired: 1 in, 9 out]
      n231 = call <vilib>:"WPI_RobotDriveTankDrive.vi"("Right axis value"=w296, "Left axis value"=w297, "RobotDriveDevRef"=w301) -> ("Motor Values"=w300:dbl[])  [unwired: 6 in, 2 out]
      n232 = call-poly <vilib>:"NT Write Value.vi"("Numeric Array"=w300, "Name"="RobotDrive Motors") -> ()  [unwired: 9 in, 1 out]
    }
    frame Disabled {
    }
  }
  n233 = case shown="False" w11 {
    frame False {
      n234 = global read "Robot Global Data.vi" "ALTURA MEDIA"() -> (w308:bool)
      n235 = global read "Robot Global Data.vi" "ESQ/DIR"() -> (w302:dbl)
      n236 = Multiply(x=145.0 ("t"), y=w302) -> (x*y=w303:dbl)
      n237 = Select(t=1190.0, s=w308, f=1900.0) -> (s? t:f=w307:dbl)
      n238 = global write "Robot Global Data.vi" "ALTURA ENTREGA"(w307) -> ()
      n239 = global write "Robot Global Data.vi" "ANGULO ENTREGA"(w303) -> ()
    }
    frame True {
      n240 = global read "Robot Global Data.vi" "ALTURA MEDIA"() -> (w312:bool)
      n241 = global read "Robot Global Data.vi" "ESQ/DIR"() -> (w311:dbl)
      n242 = Select(t=1410.0, s=w312, f=1900.0) -> (s? t:f=w315:dbl)
      n243 = Select(t=145.0, s=w312, f=183.0) -> (s? t:f=w310:dbl)
      n244 = Multiply(x=w310, y=w311) -> (x*y=w309:dbl)
      n245 = global write "Robot Global Data.vi" "ALTURA ENTREGA"(w315) -> ()
      n246 = global write "Robot Global Data.vi" "ANGULO ENTREGA"(w309) -> ()
    }
  }
  n247 = Not And(1:w18, 2:w12) -> (0:w17:bool)
  n248 = Not(x=w43) -> (.not. x?=w42:bool)
  n249 = Not(x=w16) -> (.not. x?=w15:bool)
  n250 = disable-structure shown="Enabled" {
    frame Disabled {
    }
    frame Enabled {
      n251 = call <vilib>:"WPI_CompressorRefNum Registry Get.vi"("refnum name"="Compressor") -> ("error out"=w325:errorcluster, "CompressorDevRef"=w324:T22)  [unwired: 9 in]
      n252 = call <vilib>:"WPI_CompressorGetEnableState.vi"("error in (no error)"=w325, "CompressorDevRef"=w324) -> ("error out"=w323:errorcluster, "Compressor Running"=→"Compressor Running":bool, "Enabled"=→"Enable":bool, "CompressorDevRef"=w322:T22)  [unwired: 6 in]
      n253 = call <vilib>:"WPI_CompressorRefNum Registry Set.vi"("error in (no error)"=w323, "refnum name"="Compressor", "CompressorDevRef"=w322) -> ()  [unwired: 7 in, 2 out]
    }
  }
  n254 = case shown="\"MANCHE\", Default" enum16{"MANCHE", "PID"}."MANCHE" {
    tunnel: [w327 w329] -> w64
    tunnel: [w326 w328] -> w63
    frame "MANCHE", Default {
      n255 = global read "Robot Global Data.vi" "MANCHE1"() -> (w327:dbl)
      n256 = global read "Robot Global Data.vi" "MANCHE2"() -> (w326:dbl)
    }
    frame "PID" {
      n257 = global read "Robot Global Data.vi" "SAÍDA PID ESQUERDO"() -> (w328:dbl)
      n258 = global read "Robot Global Data.vi" "SAÍDA PID DIREITO"() -> (w329:dbl)
    }
  }
  n259 = Greater?(x=w46, y=1400.0) -> (0:w44:bool)
  n260 = And(x=w42, y=w44) -> (x .and. y?=w41:bool)
  n261 = Compound Arithmetic op=AND(w17, w15, w14) -> (w13:bool)
  n262 = case shown="True" FALSE {
    frame False {
    }
    frame True {
      n263 = call <vilib>:"WPI_EncoderRefNum Registry Get.vi"("refnum name"="Encoder garra elv.") -> ("error out"=w331:errorcluster, "EncoderDevRef"=w330:T9)  [unwired: 9 in]
      n264 = call <vilib>:"WPI_EncoderReset.vi"("error in (no error)"=w331, "EncoderDevRef"=w330) -> ()  [unwired: 8 in, 2 out]
    }
  }
  n265 = case shown="True" w41 {
    frame False {
    }
    frame True {
      n266 = global read "Robot Global Data.vi" "DISCO"() -> (w333:bool)
      n267 = global read "Robot Global Data.vi" "DISCO"() -> (w334:bool)
      n268 = case shown="True" w333 {
        frame False {
        }
        frame True {
          n269 = global write "Robot Global Data.vi" "VELOCIDADE GARRA FRENTE"(-0.6 ("VELOCIDADE GARRA FRENTE")) -> ()
        }
      }
      n270 = case shown="True" w334 {
        frame False {
        }
        frame True {
          n271 = global write "Robot Global Data.vi" "VELOCIDADE GARRA FRENTE"(0.6 ("VELOCIDADE GARRA FRENTE")) -> ()
        }
      }
    }
  }
  n272 = case shown="2" 0 {
    frame 0, Default {
    }
    frame 1 {
      n273 = global write "Robot Global Data.vi" "POSI敲O"(0.0 ("f")) -> ()
    }
    frame 2 {
      n274 = global write "Robot Global Data.vi" "POSI敲O"(38.0 ("f")) -> ()
    }
    frame 4 {
      n275 = global write "Robot Global Data.vi" "POSI敲O"(145.0 ("f")) -> ()
    }
    frame 8 {
      n276 = global write "Robot Global Data.vi" "POSI敲O"(835.0 ("f")) -> ()
    }
  }
  n277 = case shown="True" w13 {
    tunnel: w12 -> [_ w342]
    frame False {
    }
    frame True {
      n278 = Not(x=w342) -> (.not. x?=w341:bool)
      n279 = global write "Robot Global Data.vi" "PROCESSO"(TRUE ("PROCESSO")) -> ()
      n280 = case shown="True" w342 {
        frame False {
          n281 = global write "Robot Global Data.vi" "POSI敲O DE PEGAR"(1103.0 ("f")) -> ()
          n282 = global write "Robot Global Data.vi" "COLUNA"(0.0 ("COLUNA")) -> ()
          n283 = global write "Robot Global Data.vi" "LINHA"(1.0 ("LINHA")) -> ()
        }
        frame True {
          n284 = global write "Robot Global Data.vi" "POSI敲O DE PEGAR"(1065.0 ("t")) -> ()
          n285 = global write "Robot Global Data.vi" "COLUNA"(0.0 ("COLUNA")) -> ()
          n286 = global write "Robot Global Data.vi" "LINHA"(0.0 ("LINHA")) -> ()
        }
      }
      n287 = global write "Robot Global Data.vi" "PEGOU BOLA"(w341) -> ()
    }
  }
  n288 = call-poly <vilib>:"NT Read Value.vi"("Name"="DB/Button 0" ("refnum name")) -> ("Boolean"=→"Sample Boolean 0":bool)  [unwired: 9 in, 1 out]
  n289 = call-poly <vilib>:"NT Read Value.vi"("Name"="DB/Slider 0" ("refnum name")) -> ("Numeric"=→"Sample Slider 0":dbl)  [unwired: 9 in, 1 out]
  n290 = call-poly <vilib>:"NT Read Value.vi"("Name"="DB/Button 1" ("refnum name")) -> ("Boolean"=→"Sample Boolean 1":bool)  [unwired: 9 in, 1 out]
  n291 = call <vilib>:"WPI_DriverStationReport Robot Code State.vi"("TeleOp"=TRUE ("Autonomous")) -> ()  [unwired: 10 in, 1 out]
  n292 = call <vilib>:"WPI_RobotDriveRefNum Registry Get.vi"("refnum name"="DRIVE MOTORS") -> ("RobotDriveDevRef"=w127:T17)  [unwired: 1 in, 9 out]
  n293 = Unbundle By Name("Match Info") -> ()  [unwired: 1 out]
  n294 = call <vilib>:"WPI_RobotDriveTankDrive.vi"("Right axis value"=w63, "Left axis value"=w64, "RobotDriveDevRef"=w127) -> ("Motor Values"=w126:dbl[])  [unwired: 6 in, 2 out]
  n295 = call-poly <vilib>:"NT Write Value.vi"("Numeric Array"=w126, "Name"="RobotDrive Motors") -> ()  [unwired: 9 in, 1 out]
